vi "ParseCommaSeparatedList.vi"(11 "List":string) -> (3 "Array":string[](array[string]))   [LabVIEW 2017]
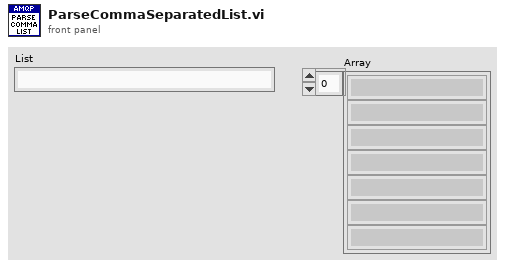
[diagram p1: front panel]
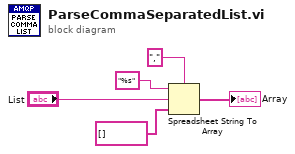
[diagram p0: block diagram]
diagram:
  n1 = Spreadsheet String To Array(delimiter (Tab)=",", format string="%s", spreadsheet string="List", array type (2D Dbl)=string[] []) -> (array=→"Array":string[])
